vi "APDM Get Device ID List.vi"(0 "APDM Context":T1={"APDM Context ID"=0, "Gyro Mode"="", "Log Data"=FALSE, "Log File"=refnum, "Gyro Record Log"=refnum, "Gyro CMD Log"=refnum, "L Opal SN"=0, "R Opal SN"=0, "Access Point ID"=0, "Left Gyro Sim Data"=path "C:/Users/jfalesi/Desktop/CP FES Walking Code/Original/Ahad Vi/CP Code/Offline data/TD_7_Raw_R.txt", "Right Gyro Sim Data"=path "C:/Users/jfalesi/Desktop/CP FES Walking Code/Original/Ahad Vi/CP Code/Offline data/TD_7_Raw_R.txt", "Sampling Rate"=0.0, "Gyro Sim Time Array"=[], "Missed Gyro Count"=0.0}, 1 "error in (no error)":errorcluster) -> (2 "APDM Context":T1={"APDM Context ID"=0, "Gyro Mode"="", "Log Data"=FALSE, "Log File"=refnum, "Gyro Record Log"=refnum, "Gyro CMD Log"=refnum, "L Opal SN"=0, "R Opal SN"=0, "Access Point ID"=0, "Left Gyro Sim Data"=path "C:/Users/jfalesi/Desktop/CP FES Walking Code/Original/Ahad Vi/CP Code/Offline data/TD_7_Raw_R.txt", "Right Gyro Sim Data"=path "C:/Users/jfalesi/Desktop/CP FES Walking Code/Original/Ahad Vi/CP Code/Offline data/TD_7_Raw_R.txt", "Sampling Rate"=0.0, "Gyro Sim Time Array"=[], "Missed Gyro Count"=0.0}, 3 "Device List":u32[](array[numeric])=[1510, 1801], 4 "error out":errorcluster)   [LabVIEW 2019]
uses:
  Controls/APDM Context Cluster.ctl
  Lee Lab/CP FES Walking 2018/Code/Working/LabVIEW/apdm.dll
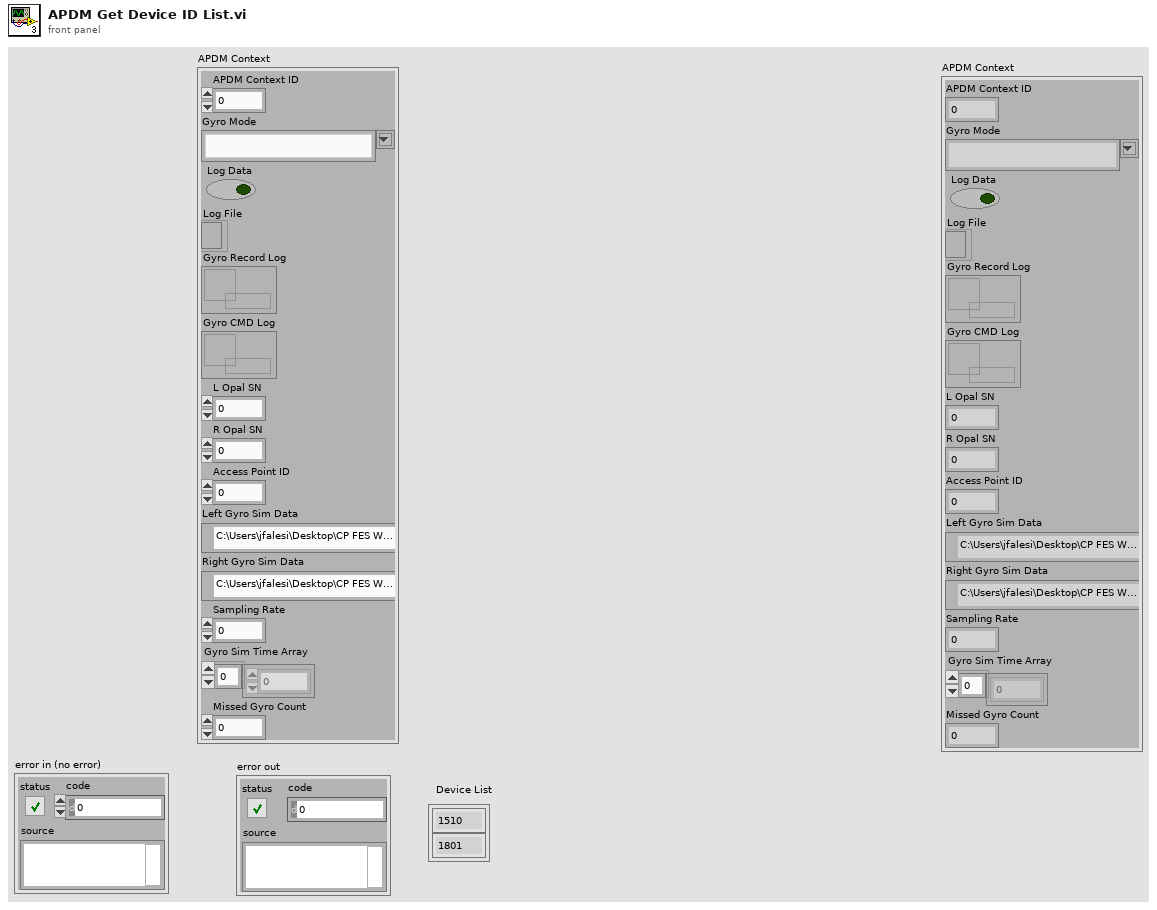
[diagram p1: front panel]
types:
  T1 = typedef "APDM Context Cluster.ctl" = cluster{"APDM Context ID":u32, "Gyro Mode":string, "Log Data":bool, "Log File":refnum<file>, "Gyro Record Log":refnum<queue>, "Gyro CMD Log":refnum<queue>, "L Opal SN":u32, "R Opal SN":u32, "Access Point ID":u32, "Left Gyro Sim Data":path, "Right Gyro Sim Data":path, "Sampling Rate":dbl, "Gyro Sim Time Array":dbl[], "Missed Gyro Count":dbl}
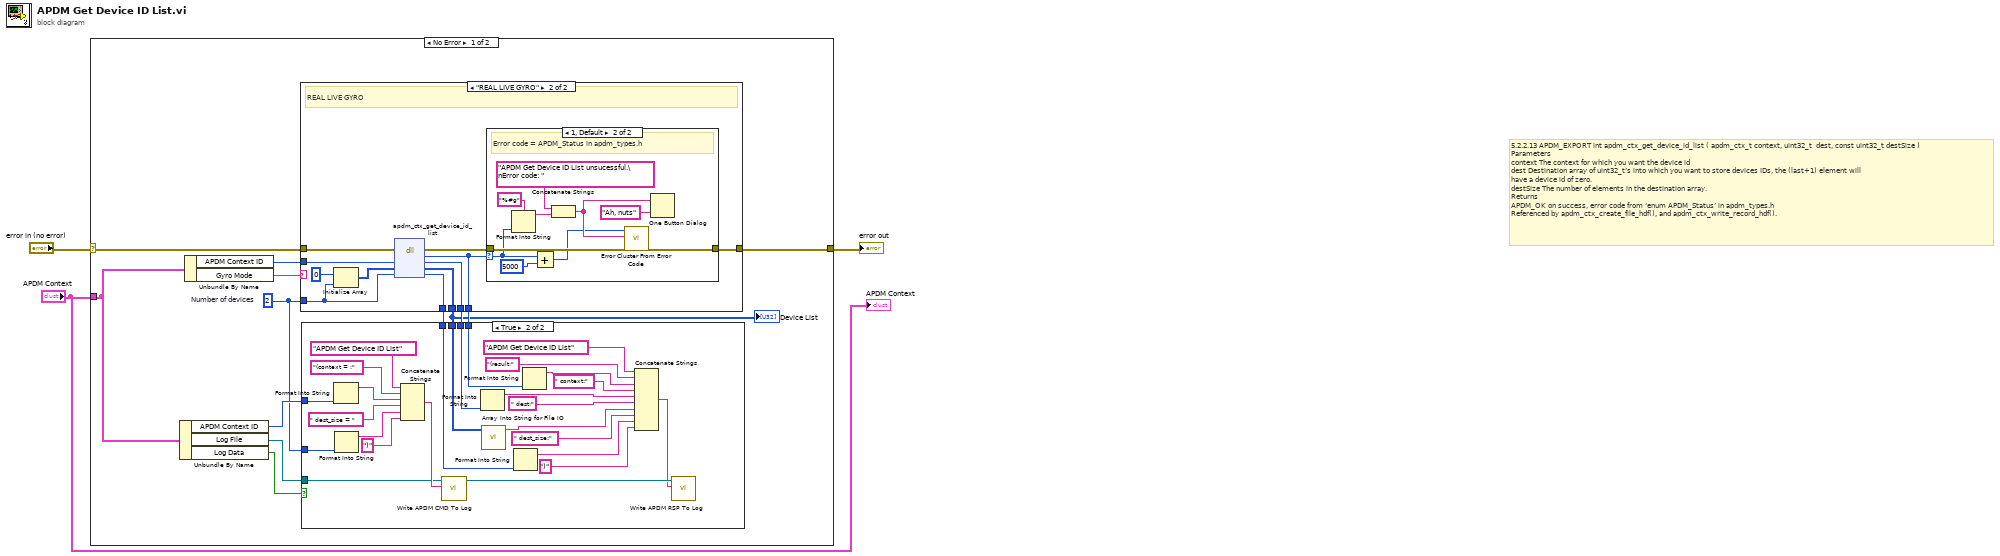
[diagram p0: block diagram]
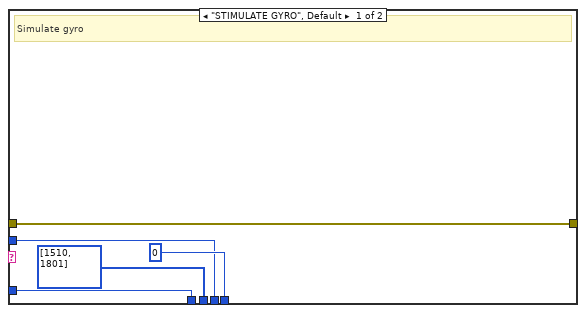
[diagram p3: hidden frame]
diagram:
  # "5.2.2.13 APDM_EXPORT int apdm_ctx_get_device_id_list ( apdm_ctx_t context, uint32_t  dest, const uint32_t destSize )\nParameters\ncontext The context for which you want the device id\ndest Destination array of uint32_t’s into which you want to store devices IDs, the (last+1) element will\nhave a device id of zero.\ndestSize The number of elements in the destination array.\nReturns\nAPDM_OK on success, error code from ’enum APDM_Status’ in apdm_types.h\nReferenced by apdm_ctx_create_file_hdf(), and apdm_ctx_write_record_hdf()."
  n1 = case shown="No Error" "error in (no error)" {
    selector: "error in (no error)" -> [w12 w70]
    tunnel: [w7 w70] -> w3
    tunnel: "APDM Context" -> [w4 _]
    frame No Error {
      w9 = 2  # Number of devices
      n2 = Unbundle By Name(w4) -> ("APDM Context ID"=w11:u32, "Log File"=w10:refnum<file>, "Log Data"=w6:bool)
      n3 = Unbundle By Name(w4) -> ("APDM Context ID"=w14:u32, "Gyro Mode"=w13:string)
      n4 = case shown="\"REAL LIVE GYRO\"" w13 {
        tunnel: w14 -> [w43 w57]
        tunnel: w12 -> [w45 w58]
        tunnel: [w43 w56] -> w16
        tunnel: [u32[] [1510, 1801] ("Device List 2") w55] -> w5
        tunnel: [0 w54] -> w15
        tunnel: w9 -> [w46 w51]
        tunnel: [w46 w50] -> w8
        tunnel: [w45 w48] -> w7
        frame "STIMULATE GYRO", Default {
          # "Simulate gyro"
        }
        frame "REAL LIVE GYRO" {
          # "REAL LIVE GYRO"
          n5 = Initialize Array(u32 0, w51) -> (w52:u32[])
          n6 = dll-call lib="C:/Users/jfalesi/Dropbox/Lee Lab/CP FES Walking 2018/Code/Working/LabVIEW/apdm.dll" fn="apdm_ctx_get_device_id_list"(error in=w58, "Context"=w57, "Dest"=w52, "dest size"=w51) -> (error out=w49:errorcluster, "return type"=w54:i32, "Context"=w56:u32, "Dest"=w55:u32[], "dest size"=w50:i32)  [unwired: 2 in, 1 out]
          n7 = case shown="1, Default" w54 {
            selector: w54 -> [_ w62]
            tunnel: w49 -> [w59 w66]
            tunnel: [w59 w65] -> w48
            frame 0 {
              # "No error"
            }
            frame 1, Default {
              # "Error code = APDM_Status in apdm_types.h"
              n8 = Format Into String(format string="%#g", w62) -> (resulting string=w68:string)  [unwired: 2 in, 1 out]
              n9 = Add(x=w62, y=5000) -> (x+y=w60:i32)
              n10 = Concatenate Strings("APDM Get Device ID List unsucessful.\nError code: " ("message"), w68) -> (w64:string)
              n11 = call <vilib>:"Error Cluster From Error Code.vi"("error in (no error)"=w66, "error message (\"\")"=w64, "error code (0)"=w60) -> ("error out"=w65:errorcluster)  [unwired: 6 in]
              n12 = One Button Dialog(message=w64, button name ("OK")="Ah, nuts") -> ()  [unwired: 1 out]
            }
          }
        }
      }
      "Device List" <- w5
      n13 = case shown="True" w6 {
        tunnel: w16 -> [_ w29]
        tunnel: w5 -> [_ w28]
        tunnel: w15 -> [_ w26]
        tunnel: w10 -> [_ w20]
        tunnel: w11 -> [_ w19]
        tunnel: w9 -> [_ w18]
        tunnel: w8 -> [_ w17]
        frame False {
        }
        frame True {
          n14 = Format Into String(w19) -> (resulting string=w39:string)  [unwired: 3 in, 1 out]
          n15 = Format Into String(w18) -> (resulting string=w37:string)  [unwired: 3 in, 1 out]
          n16 = Concatenate Strings("APDM Get Device ID List" ("Log Item"), "(context = :" ("string"), w39, " dest_size = " ("string"), w37, ")" ("string")) -> (w22:string)
          n17 = call "Write APDM CMD To Log.vi"("Log Item"=w22, "Byte Stream File in"=w20) -> ("Byte Stream File out"=w42:refnum<file>)  [unwired: 8 in, 1 out]
          n18 = Format Into String(w29) -> (resulting string=w34:string)  [unwired: 3 in, 1 out]
          n19 = call "Array Into String for File IO.vi"("Array"=w28) -> ("result string"=w21:string)  [unwired: 10 in]
          n20 = Format Into String(w17) -> (resulting string=w31:string)  [unwired: 3 in, 1 out]
          n21 = Format Into String(w26) -> (resulting string=w25:string)  [unwired: 3 in, 1 out]
          n22 = Concatenate Strings("APDM Get Device ID List" ("Log Item"), "(result:" ("string"), w25, " context:" ("string"), w34, " dest:" ("string"), w21, " dest_size:" ("string"), w31, ")" ("string")) -> (w23:string)
          n23 = call "Write APDM RSP To Log.vi"("Log Item"=w23, "Byte Stream File in"=w42) -> ()  [unwired: 9 in, 1 out]
        }
      }
    }
    frame Error {
    }
  }
  "error out" <- w3
  "APDM Context" <- "APDM Context"
